vi "Sysdef.SimpleExport(subSection).vi"(8 "error in (no error)":errorcluster, 11 "ID":u64) -> (0 "error out":errorcluster, 2 "Exported Section":T1 {"Tree"."Properties"."Type" items=["K_STRING", "K_BOOL", "K_I32", "K_U32", "K_DOUBLE", "K_U64", "K_VARIANT", "K_DEPENDENTFILE", "K_DEPENDENTNODE", "K_DATASOURCENODE", "K_U16", "K_DBLARR", "K_U32ARR", "K_I32ARR", "K_STRINGARR", "K_DICTIONARY", "K_DICTIONARYARR"]}, 3 "ID out":u64)   [LabVIEW 2020, in "ImportExport.lvlib"]
doc: "Uses the NI VeriStand .NET API to save the Custom Device Hierarchy (Sections, Channels, Waveforms) as well as its Items Properties into a cluster."
uses:
  ImportExport.lvlib
  <vilib>/NI/NI VeriStand Advanced SysDef API/_Types/SysDef.Export.subSection.ctl
  <vilib>/NI/NI VeriStand Advanced SysDef API/_Types/TreeItem.ctl
  <vilib>/NI/NI VeriStand Advanced SysDef API/_Types/TreeItem.Info.ctl
  <vilib>/NI VeriStand/Custom Device API/Custom Device Channel.ctl
  <vilib>/NI VeriStand/Custom Device API/Custom Device Channel Type.ctl
  <vilib>/NI VeriStand/Custom Device API/Custom Device Waveform.ctl
  <vilib>/NI VeriStand/Custom Device API/Custom Device Waveform DataType.ctl
  <vilib>/NI/NI VeriStand Advanced SysDef API/_Types/TreeItem.Property.ctl
  NationalInstruments.VeriStand.SystemDefinitionAPI
  <vilib>/NI/NI VeriStand Advanced SysDef API/SysDef API/Advanced System Definition.lvlib
  <vilib>/NI VeriStand/Custom Device API/Custom Device API.lvlib
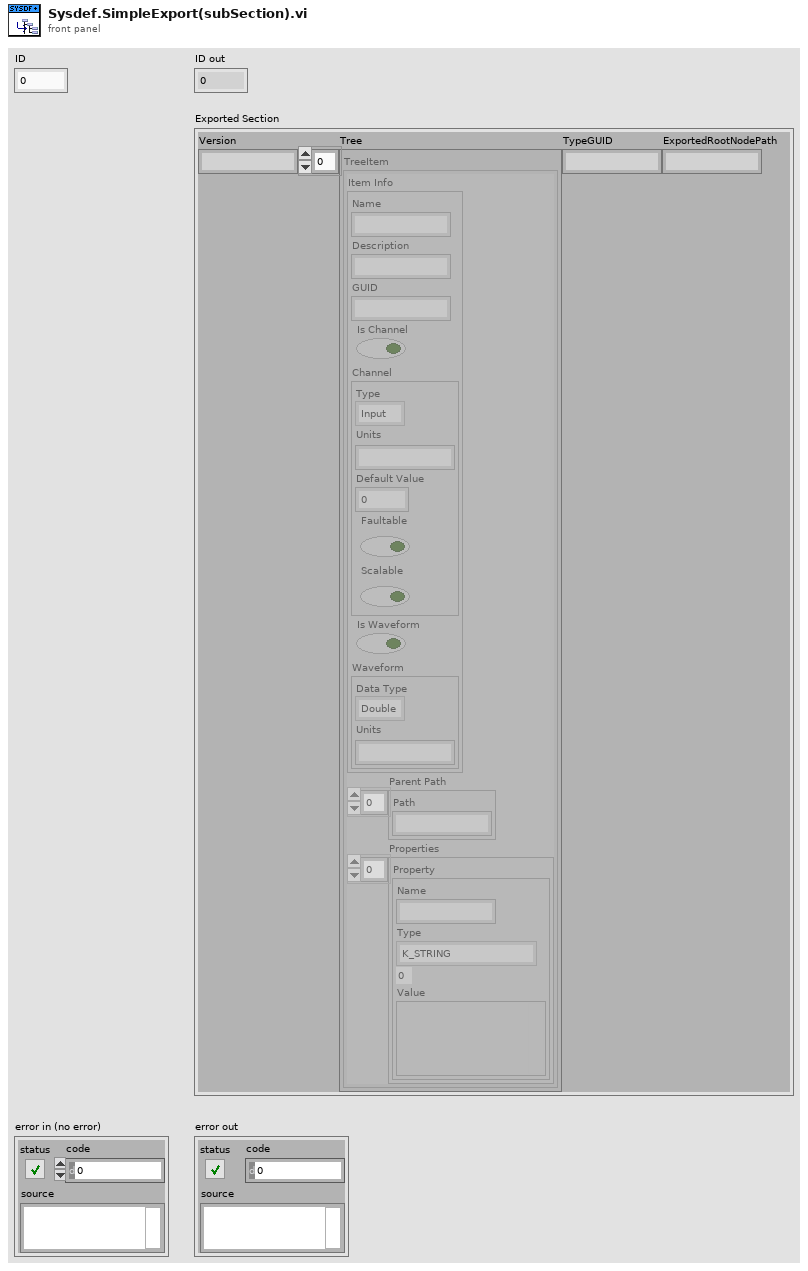
[diagram p1: front panel]
types:
  T1 = typedef "Advanced System Definition.lvlib/SysDef.Export.subSection.ctl" = cluster{"Version":string, "Tree":T2[], "TypeGUID ":string, "ExportedRootNodePath":string}
  T2 = typedef "Advanced System Definition.lvlib/TreeItem.ctl" = cluster{"Item Info":T3, "Parent Path":string[], "Properties":T8[]}
  T3 = typedef "Advanced System Definition.lvlib/TreeItem.Info.ctl" = cluster{"Name":string, "Description":string, "GUID":string, "Is Channel":bool, "Channel":T4, "Is Waveform":bool, "Waveform":T6}
  T4 = typedef "Custom Device API.lvlib/Custom Device Channel.ctl" = cluster{"Type":T5, "Units":string, "Default Value":dbl, "Faultable":bool, "Scalable":bool}
  T5 = typedef "Custom Device API.lvlib/Custom Device Channel Type.ctl" = enum16{"Input", "Output"}
  T6 = typedef "Custom Device API.lvlib/Custom Device Waveform.ctl" = cluster{"Data Type":T7, "Units":string}
  T7 = typedef "Custom Device API.lvlib/Custom Device Waveform DataType.ctl" = enum16{"Double", "Complex Double"}
  T8 = typedef "Advanced System Definition.lvlib/TreeItem.Property.ctl" = cluster{"Name":string, "Type":i32, "Value":variant}
  T9 = typedef "Custom Device API.lvlib/Custom Device Item Ref.ctl" = u64
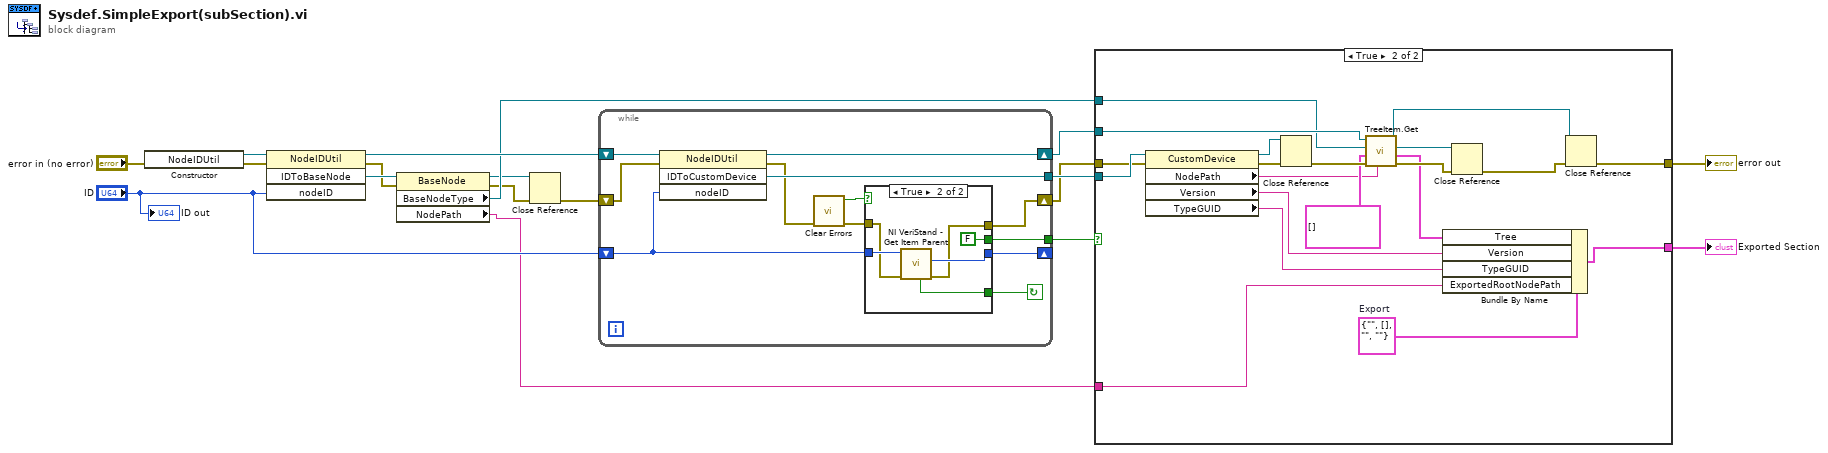
[diagram p0: block diagram]
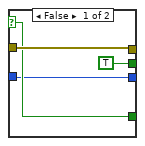
[diagram p2: hidden frame]
diagram:
  n1 = constructor class="NodeIDUtil"(error in="error in (no error)") -> (reference out=w13:refnum<k24>, error out=w12:errorcluster)  [unwired: 2 in, 1 out]
  n2 = invoke class="NodeIDUtil" method="IDToBaseNode"(reference=w13, error in=w12, "nodeID"="ID") -> (reference out=w11:refnum<k24>, error out=w9:errorcluster, "IDToBaseNode"=w10:refnum<k24>)  [unwired: 1 in, 1 out]
  n3 = property class="BaseNode"(reference=w10, error in=w9) -> (reference out=w5:refnum<k24>, error out=w6:errorcluster, "BaseNodeType"=w8:refnum<k24>, "NodePath"=w2:string)
  n4 = Close Reference(reference=w5, error in (no error)=w6) -> (error out=w4:errorcluster)
  n5 = while {
    tunnel: [w30] -> w18
    shift-right: [w29] -> w16
    shift-left: w11 -> [w28]
    shift-right: [w20] -> w3
    shift-left: w4 -> [w26]
    shift-right: [w22] -> _
    shift-left: "ID" -> [w23]
    tunnel: [w19] -> w1
    stop <- w21 continue-if-true
    n6 = invoke class="NodeIDUtil" method="IDToCustomDevice"(reference=w28, error in=w26, "nodeID"=w23) -> (reference out=w29:refnum<k24>, error out=w27:errorcluster, "IDToCustomDevice"=w30:refnum<k24>)  [unwired: 1 in, 1 out]
    n7 = call <vilib>:"Clear Errors.vi"("error in (no error)"=w27) -> ("error out"=w24:errorcluster, "specific error cleared?"=w25:bool)  [unwired: 5 in]
    n8 = case shown="True" w25 {
      selector: w25 -> [w33 _]
      tunnel: w24 -> [w34 w37]
      tunnel: w23 -> [w32 w40]
      tunnel: [w32 w39] -> w22
      tunnel: [w33 w38] -> w21
      tunnel: [w34 w36] -> w20
      tunnel: [TRUE FALSE] -> w19
      frame False {
      }
      frame True {
        n9 = call <vilib>:"NI VeriStand - Get Item Parent.vi"("error in (no error)"=w37, "Item Ref in"=w40) -> ("error out"=w36:errorcluster, "Parent Ref"=w39:T9, "Found"=w38:bool)  [unwired: 6 in, 1 out]
      }
    }
  }
  n10 = case shown="True" w1 {
    tunnel: w18 -> [_ w61]
    tunnel: w16 -> [_ w57]
    tunnel: [w41 w53] -> w15
    tunnel: [_ w49] -> w14
    tunnel: w8 -> [_ w44]
    tunnel: w3 -> [w41 w43]
    tunnel: w2 -> [_ w42]
    frame False {
    }
    frame True {
      w46 = T1 {"Version"="", "Tree"=[], "TypeGUID "="", "ExportedRootNodePath"=""}  # Export
      n11 = property class="CustomDevice"(reference=w61, error in=w43) -> (reference out=w58:refnum<k24>, error out=w60:errorcluster, "NodePath"=w47:string, "Version"=w50:string, "TypeGUID"=w45:string)
      n12 = Close Reference(reference=w58, error in (no error)=w60) -> (error out=w59:errorcluster)
      n13 = call <vilib>:"TreeItem.Get.vi"("Custom Device Path"=w47, "error in (no error)"=w59, "Tree"=T2[] [], "BaseNode Ref"=w44, "NodeIDUtil Ref"=w57) -> ("error out"=w55:errorcluster, "Tree"=w48:T2[], "BaseNode Ref out"=w56:refnum<k24>, "NodeIDUtil Ref out"=w52:refnum<k24>)  [unwired: 3 in]
      n14 = Bundle By Name(cluster=w46, "Tree"=w48, "Version"=w50, "TypeGUID"=w45, "ExportedRootNodePath"=w42) -> (w49:T1)
      n15 = Close Reference(reference=w56, error in (no error)=w55) -> (error out=w54:errorcluster)
      n16 = Close Reference(reference=w52, error in (no error)=w54) -> (error out=w53:errorcluster)
    }
  }
  "error out" <- w15
  "Exported Section" <- w14
  "ID out" <- "ID"
